vi "Suite.vi"(8 "error in (no error)":errorcluster, 10 "LUnit Test Suite in":refnum<class "Test Suite.lvclass">, 11 "LUnit Test Case in":refnum<class "LUnit Inheriting Test Case.lvclass">) -> (0 "error out":errorcluster, 2 "LUnit Test Suite Out":refnum<class "Test Suite.lvclass">, 3 "LUnit Test Case out":refnum<class "LUnit Inheriting Test Case.lvclass">)   [LabVIEW 2020, in "LUnit Inheriting Test Case.lvclass"]
uses:
  LUnit Inheriting Test Case.lvclass
  C:/Program Files (x86)/National Instruments/LabVIEW 2020/vi.lib/Astemes/LUnit/Test Case.lvclass
  C:/Program Files (x86)/National Instruments/LabVIEW 2020/vi.lib/Astemes/LUnit/LUnit Runnable.lvclass
  <vilib>/Astemes/LUnit/Test Suite.lvclass
  <vilib>/Astemes/LUnit/Test Case.lvclass/Test Case.ctl
  <vilib>/Utility/LVClass/Get LV Class Name.vi
  <vilib>/Astemes/LUnit/Test Case.lvclass
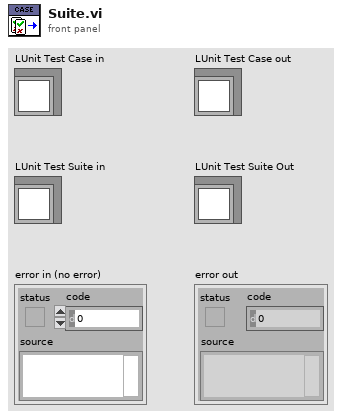
[diagram p1: front panel]
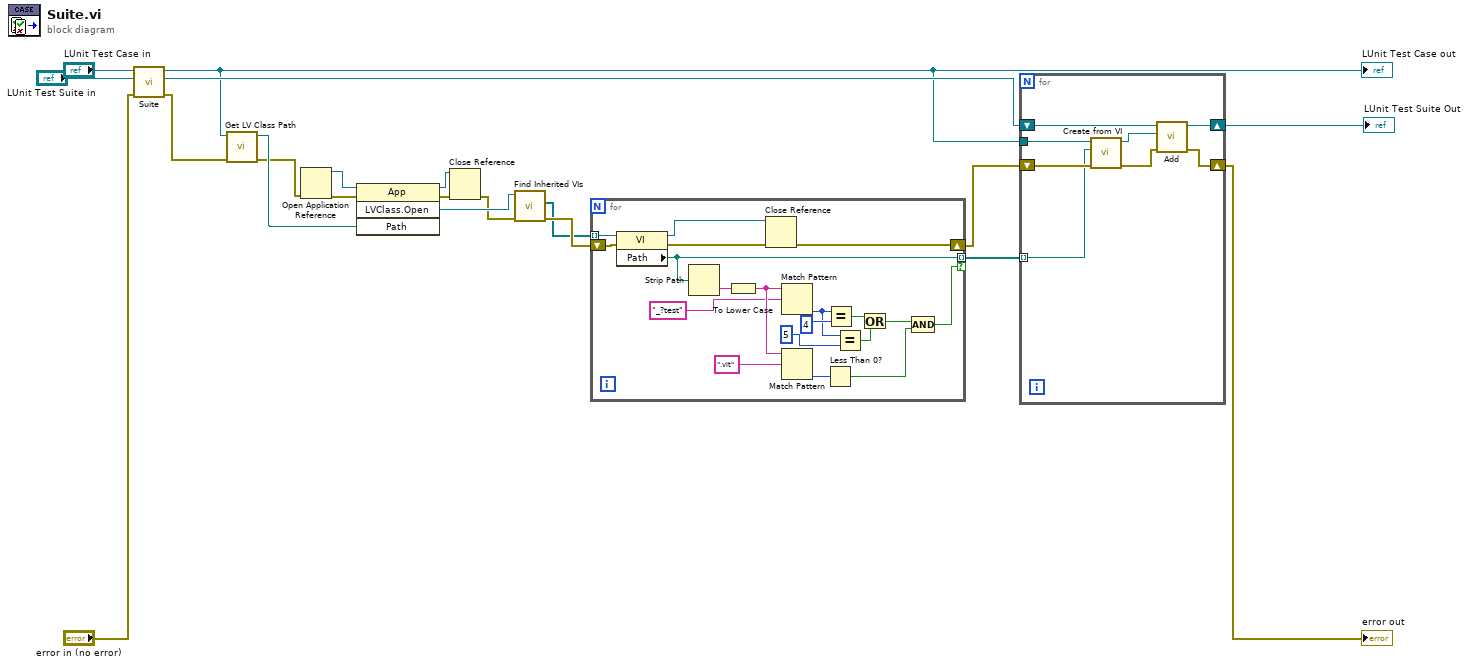
[diagram p0: block diagram]
diagram:
  n1 = call-parent "Suite.vi"("error in (no error)"="error in (no error)", "LUnit Test Suite in"="LUnit Test Suite in", "Test Case Class in"="LUnit Test Case in") -> ("error out"=w5:errorcluster, "LUnit Test Suite Out"=w4:refnum<class "Test Suite.lvclass">, "LUnit Test Case out"=w2:refnum<class "LUnit Inheriting Test Case.lvclass">)  [unwired: 6 in]
  "LUnit Test Case out" <- w2
  n2 = call <vilib>:"Get LV Class Path.vi"("error in (no error)"=w5, "object"=w2) -> ("error out"=w9:errorcluster, "class path"=w10:path)  [unwired: 8 in]
  n3 = Open Application Reference(8:w9) -> (0:w18:errorcluster, 3:w19:refnum<vi>)  [unwired: 3 in]
  n4 = invoke class="App" method="LVClass.Open"(reference=w19, error in=w18, "Path"=w10) -> (reference out=w15:refnum<vi>, error out=w17:errorcluster, "LVClass.Open"=w14:refnum<vi>)  [unwired: 1 in, 1 out]
  n5 = Close Reference(reference=w15, error in (no error)=w17) -> (error out=w11:errorcluster)
  n6 = call "Find Inherited VIs.vi"("error in (no error)"=w11, "LVClassLibrary in"=w14) -> ("error out"=w13:errorcluster, "Inherited Dynamic Member VIs"=w3:refnum<vi>[])  [unwired: 8 in]
  n7 = for {
    tunnel: w3 -> [w39] mode=indexing
    tunnel: [w34] -> w16 mode=indexing if=w29
    shift-right: [w36] -> w12
    shift-left: w13 -> [w38]
    n8 = property class="VI"(reference=w39, error in=w38) -> (reference out=w35:refnum<vi>, error out=w37:errorcluster, "Path"=w34:path)
    n9 = Strip Path(path=w34) -> (name=w33:string)  [unwired: 1 out]
    n10 = To Lower Case(string=w33) -> (all lower case string=w32:string)
    n11 = Close Reference(reference=w35, error in (no error)=w37) -> (error out=w36:errorcluster)
    n12 = Match Pattern(string=w32, regular expression="_?test") -> (offset past match=w26:i32)  [unwired: 1 in, 3 out]
    n13 = Match Pattern(string=w32, regular expression=".vit") -> (offset past match=w30:i32)  [unwired: 1 in, 3 out]
    n14 = Less Than 0?(x=w30) -> (x < 0?=w28:bool)
    n15 = Equal?(x=w26, y=4) -> (x = y?=w24:bool)
    n16 = Equal?(x=w26, y=5) -> (x = y?=w21:bool)
    n17 = Or(x=w24, y=w21) -> (x .or. y?=w22:bool)
    n18 = Compound Arithmetic op=AND(w22, w28) -> (w29:bool)
  }
  n19 = for {
    tunnel: w16 -> [w40] mode=indexing
    shift-right: [w46] -> w8
    shift-left: w4 -> [w47]
    shift-right: [w44] -> w7
    shift-left: w12 -> [w43]
    tunnel: w2 -> [w41]
    n20 = call <vilib>:"Create from VI.vi"("error in (no error)"=w43, "Test Method VI Path"=w40, "LUnit Test Case Class"=w41) -> ("error out"=w45:errorcluster, "LUnit Test Case Out"=w42:refnum<class "LUnit Inheriting Test Case.lvclass">)  [unwired: 7 in]
    n21 = call <vilib>:"Add.vi"("error in (no error)"=w45, "Runnable"=w42, "LUnit Test Suite In"=w47) -> ("error out"=w44:errorcluster, "LUnit Test Suite Out"=w46:refnum<class "Test Suite.lvclass">)  [unwired: 7 in]
  }
  "error out" <- w7
  "LUnit Test Suite Out" <- w8
